vi "Get Cache.vi"(11 "ConfigManager in":refnum<class "ConfigManager.lvclass">) -> (1 "found?":bool, 2 "Cache":refnum<class "ConfigManager.Cache.lvclass">, 3 "ConfigManager out":refnum<class "ConfigManager.lvclass">)   [LabVIEW 2013, in "SMOConfig.lvlib" / "ConfigManager.lvclass"]
uses:
  ConfigManager.lvclass
  Cache/ConfigManager.Cache.lvclass
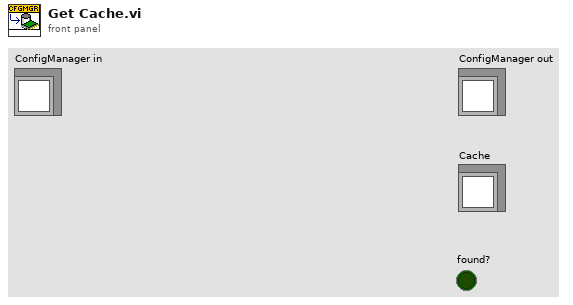
[diagram p1: front panel]
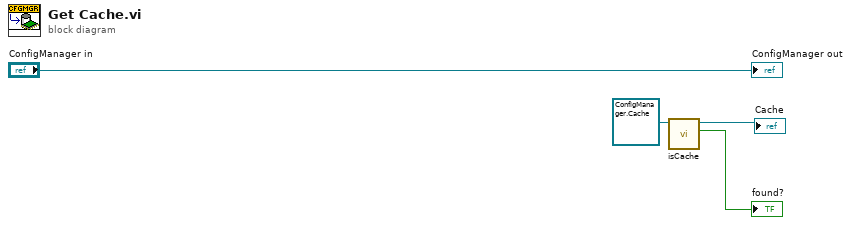
[diagram p0: block diagram]
diagram:
  n1 = call "isCache.vi"("ConfigManager.Cache in"=refnum<class "ConfigManager.Cache.lvclass"> refnum) -> ("isCache?"=→"found?":bool, "ConfigManager.Cache out"=→"Cache":refnum<class "ConfigManager.Cache.lvclass">)  [unwired: 9 in]
  "ConfigManager out" <- "ConfigManager in"
